vi "QPSK (SubVI).vi"(11 "output bit stream":i8[](array[numeric])) -> (3 "Array":cdb[](array[numeric]))   [LabVIEW 2018]
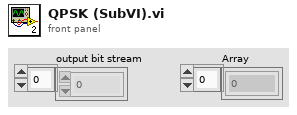
[diagram p1: front panel]
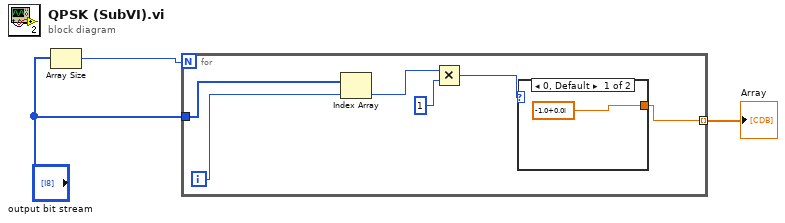
[diagram p0: block diagram]
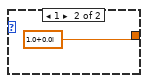
[diagram p2: hidden frame]
diagram:
  n1 = Array Size(array="output bit stream") -> (size(s)=w1:i32)
  n2 = for {
    N: w1 -> [_]
    tunnel: "output bit stream" -> [w9]
    tunnel: [w6] -> w3 mode=indexing
    i -> [w4]
    n3 = Index Array(array=w9, index=w4) -> (element=w7:i8)
    n4 = Multiply(x=w7, y=1) -> (x*y=w5:i32)
    n5 = case shown="0, Default" w5 {
      tunnel: [cdb -1.0+0.0i cdb 1.0+0.0i] -> w6
      frame 0, Default {
      }
      frame 1 {
      }
    }
  }
  "Array" <- w3
